vi "UpdateGrafica.vi"(8 "error in (no error)":errorcluster, 10 "event data":waveform(dbl), 11 "GUI SeñalActualizable in":refnum<class "GUI SeñalActualizable.lvclass">) -> (0 "error out":errorcluster, 3 "GUI SeñalActualizable out":refnum<class "GUI SeñalActualizable.lvclass">)   [LabVIEW 2020, in "GUI SeñalActualizable.lvlib" / "GUI SeñalActualizable.lvclass"]
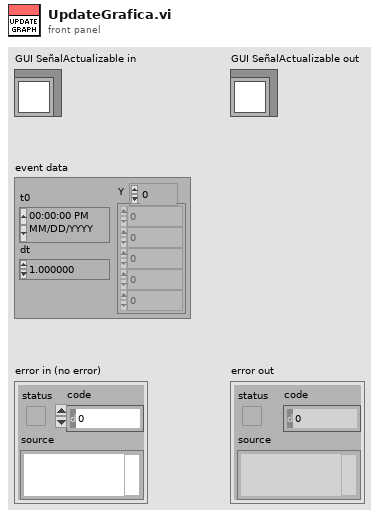
[diagram p1: front panel]
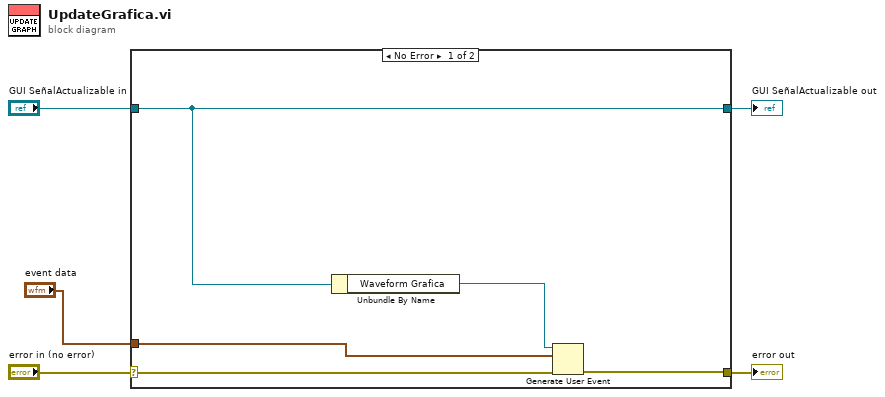
[diagram p0: block diagram]
diagram:
  n1 = case shown="No Error" "error in (no error)" {
    selector: "error in (no error)" -> [w7 w12]
    tunnel: [w8 w12] -> w4
    tunnel: [w10 w11] -> w2
    tunnel: "GUI SeñalActualizable in" -> [w10 w11]
    tunnel: "event data" -> [w6 _]
    frame No Error {
      n2 = Unbundle By Name(w10) -> ("Waveform Grafica"=w9:refnum<user-event>)
      n3 = Generate User Event(user event=w9, event data cluster=w6, error in=w7) -> (error out=w8:errorcluster)  [unwired: 1 in, 1 out]
    }
    frame Error {
    }
  }
  "error out" <- w4
  "GUI SeñalActualizable out" <- w2
